vi "Read Data From Excel.vi"() -> ()   [LabVIEW 2013]
uses:
  <vilib>/addons/_office/NI_ReportGenerationToolkit.lvlib
panel:
  out "Value2":variant
  out "x/y":dbl[](array[numeric])
  in  "Stop":string="B6"
  in  "Start":string="A1"
  out "error out":errorcluster
  in  "path":path
  in  "sheet name":string="Sheet1"
  in  "Excel.Worksheet":refnum<k7>
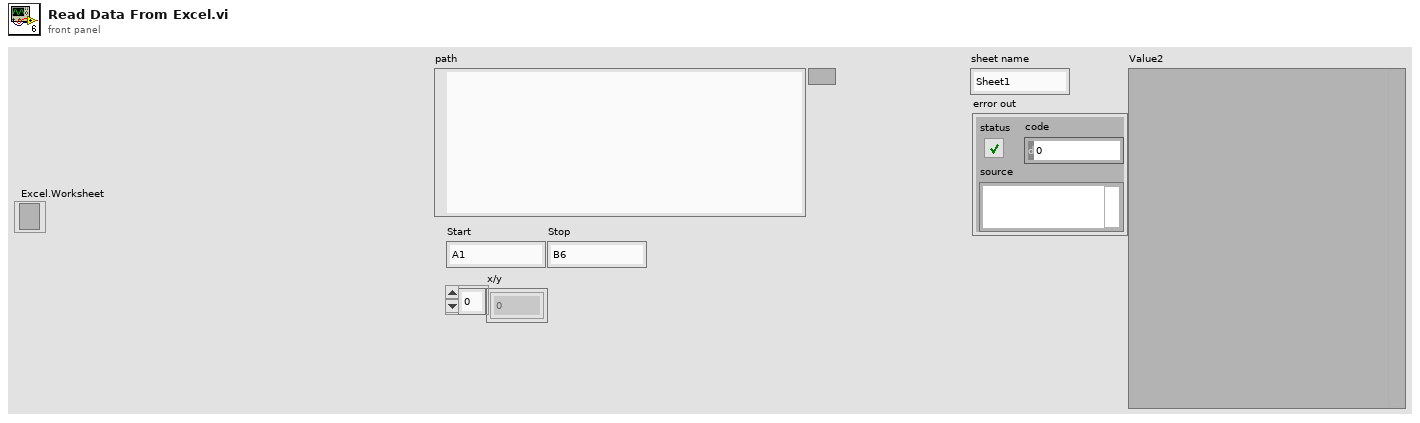
[diagram p1: front panel]
types:
  T1 = enum16{"maximized", "minimized", "normal", "no change"}
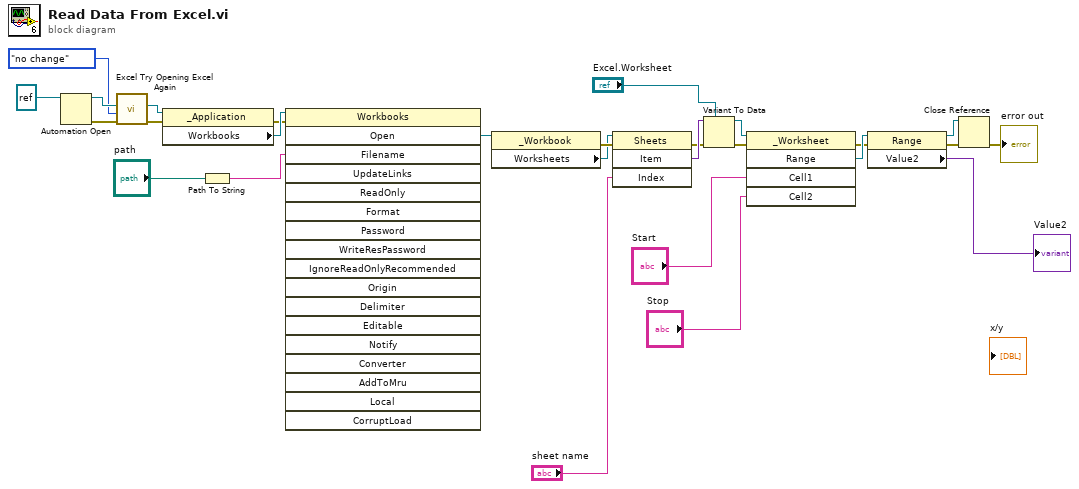
[diagram p0: block diagram]
diagram:
  n1 = Automation Open(Automation Refnum=refnum<k7> refnum ("Excel._Application")) -> (Automation Refnum=w21:refnum<k7>, error out=w23:errorcluster)  [unwired: 1 in, 2 out]
  n2 = call <vilib>:"Excel Try Opening Excel Again.vi"("error in (no error)"=w23, "window state (normal)"=T1."no change", "Excel._Application in"=w21) -> ("error out"=w22:errorcluster, "Excel._Application out"=w20:refnum<k7>)  [unwired: 3 in, 4 out]
  n3 = property class="_Application"(reference=w20, error in=w22) -> (error out=w26:errorcluster, "Workbooks"=w27:refnum<k7>)  [unwired: 1 out]
  n4 = Path To String(path="path") -> (string=w24:string)
  n5 = invoke class="Workbooks" method="Open"(reference=w27, error in=w26, "Filename"=w24) -> ("Open"=w9:refnum<k7>)  [unwired: 15 in, 17 out]
  n6 = property class="_Workbook"(reference=w9) -> (error out=w18:errorcluster, "Worksheets"=w11:refnum<k7>)  [unwired: 1 in, 1 out]
  n7 = invoke class="Sheets" method="Item"(reference=w11, error in=w18, "Index"="sheet name") -> (error out=w13:errorcluster, "Item"=w15:variant)  [unwired: 1 in, 2 out]
  n8 = Variant To Data(error in=w13, type="Excel.Worksheet", Variant=w15) -> (data=w10:refnum<k7>, error out=w14:errorcluster)
  n9 = invoke class="_Worksheet" method="Range"(reference=w10, error in=w14, "Cell1"="Start", "Cell2"="Stop") -> (error out=w16:errorcluster, "Range"=w17:refnum<k7>)  [unwired: 1 in, 3 out]
  n10 = property class="Range"(reference=w17, error in=w16) -> (reference out=w6:refnum<k7>, error out=w5:errorcluster, "Value2"=→"Value2":variant)
  n11 = Close Reference(reference=w6, error in (no error)=w5) -> (error out=→"error out":errorcluster)
